vi "CIC_downsample_reconfig.vi"(6 "Gain":fxp<+/-,32,1>=0.00390625 format="%#_32g", 7 "new rate":fxp<+,8,8>, 8 "valid in":bool, 10 "Data in":fxp<+/-,16,14>, 11 "rate change":bool) -> (0 "valid out":bool, 1 "rdy for data":bool, 2 "dout":fxp<+/-,16,14>)   [LabVIEW 2013]
uses:
  <vilib>/rvi/FXPMathLib/FxpConvert/subVIs/nifxpmath_Convert_SimConfig.ctl
  <vilib>/fxp/LVFixedPointQuantizationPolicyTypeDef.ctl
  <vilib>/fxp/LVFixedPointOverflowPolicyTypeDef.ctl
  <vilib>/rvi/FXPMathLib/FxpConvert/simVIs/DllFxpConvertTemp_sub.vi
  <vilib>/rvi/IPIntegrationNode/IPINode_Utilities/niFpgaIPINodeSimCore.vi
  <vilib>/rvi/FXPMathLib/FxpConvert/XNode/nifxpmath_Convert.xnode
  <vilib>/rvi/XilinxIP/XIPIN_XNode/niFpgaXIPIN.xnode
  C:/Users/Public/Documents/LabVIEW-proj/PXIe/Workspace/Filters/CIC_reconfig/CIC_reconfig_98CB1CAE2BB740CC8D7F2D4651806219.dll
  <vilib>/rvi/IPIntegrationNode/IPINode_Xnode/niFpgaIPINode.xnode
  <vilib>/rvi/FXPMathLib/FxpMul/XNode/nifxpmath_Multiplier.xnode
  <vilib>/rvi/FXPMathLib/sim/FxpSim.dll
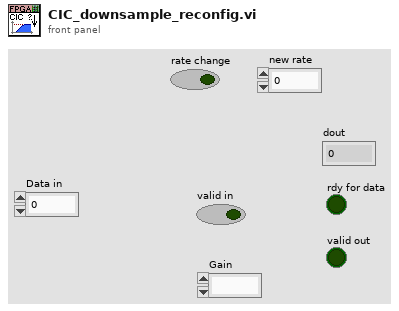
[diagram p1: front panel]
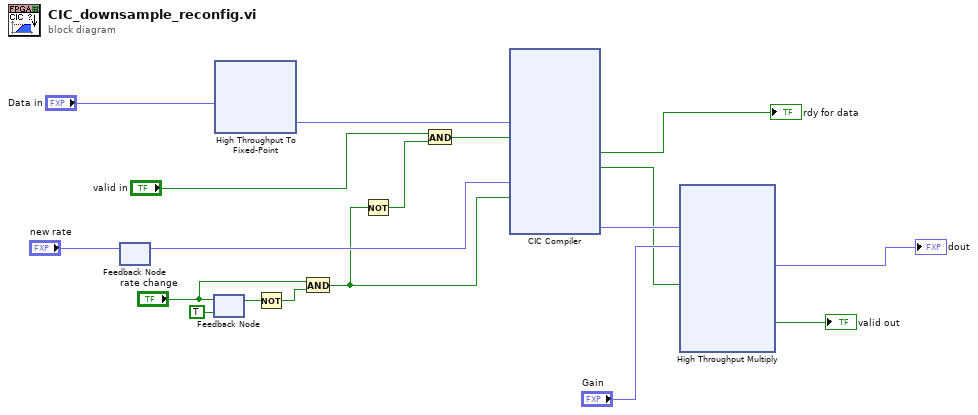
[diagram p0: block diagram]
diagram:
  n1 = feedback #1() -> (w8:fxp<+,8,8>)  [unwired: 1 in]
  n2 = feedback-in #1("new rate") -> ()
  n3 = feedback-in #2("rate change") -> ()
  n4 = feedback #2(TRUE ("rate change")) -> (w18:bool)
  n5 = xnode "High Throughput To Fixed-Point"("x"="Data in") -> ("y"=w10:fxp<+,16,16>)
  n6 = Not(x=w18) -> (.not. x?=w16:bool)
  n7 = And(x="rate change", y=w16) -> (x .and. y?=w7:bool)
  n8 = Not(x=w7) -> (.not. x?=w12:bool)
  n9 = And(x="valid in", y=w12) -> (x .and. y?=w9:bool)
  n10 = xnode ("CIC Compiler")("s_axis_data_tdata"=w10, "s_axis_data_tvalid"=w9, "s_axis_config_tdata"=w8, "s_axis_config_tvalid"=w7) -> ("s_axis_data_tready"=→"rdy for data":bool, "m_axis_data_tvalid"=w3:bool, "m_axis_data_tdata"=w6:fxp<+/-,32,32>)  [unwired: 2 in, 1 out]
  n11 = xnode ("High Throughput Multiply")("x"=w6, "y"="Gain", "input valid"=w3) -> ("x*y"=→"dout":fxp<+/-,16,14>, "output valid"=→"valid out":bool)  [unwired: 1 in, 1 out]
